vi "Timer Process.vi"(8 "error in (no error)":errorcluster, 10 "Timer Display Refnum":refnum<vi>, 11 "Background Control Queue":refnum<queue>) -> (0 "error out":errorcluster)   [LabVIEW 2015, in "Execution.lvclass"]
uses:
  Execution.lvclass
  BACKGROUND_CONTROL_MSG_TYPEDEF.ctl
panel:
  out "STOP_FLAG":bool
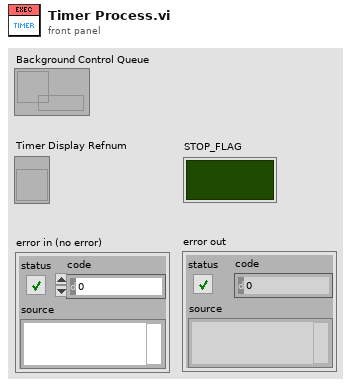
[diagram p1: front panel]
types:
  T1 = typedef "Execution.lvclass/BACKGROUND_CONTROL_MSG_TYPEDEF.ctl" = cluster{"Target":string, "Msg":string, "Data":variant}
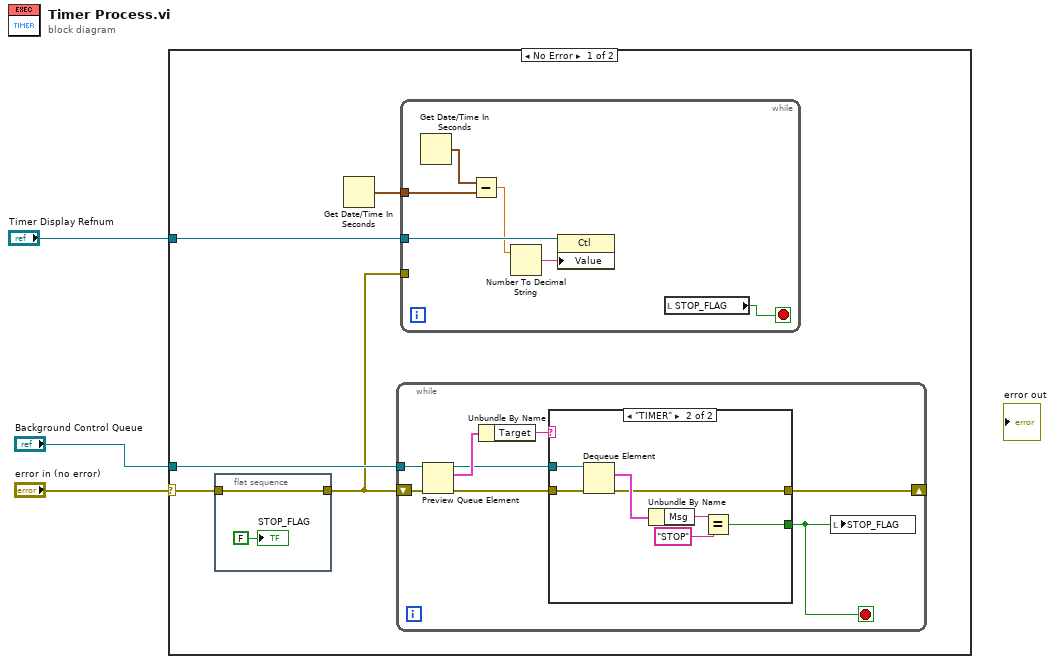
[diagram p0: block diagram]
diagram:
  n1 = case shown="No Error" "error in (no error)" {
    selector: "error in (no error)" -> [w6 _]
    tunnel: "Background Control Queue" -> [w7 _]
    tunnel: "Timer Display Refnum" -> [w4 _]
    frame No Error {
      n2 = flat-sequence {
        tunnel: w6 -> [w10]
        tunnel: [w10] -> w5
        frame #0 {
          "STOP_FLAG" <- FALSE ("STOP_FLAG")
        }
      }
      n3 = Get Date/Time In Seconds() -> (seconds since 1Jan1904=w8:timestamp)
      n4 = while {
        shift-right: [w12] -> _
        shift-left: w5 -> [w18]
        tunnel: w7 -> [w17]
        stop <- w11 stop-if-true
        n5 = Preview Queue Element(queue=w17, error in (no error)=w18) -> (queue out=w13:refnum<queue>, element=w16:T1, error out=w14:errorcluster)  [unwired: 1 in, 1 out]
        n6 = Unbundle By Name(w16) -> ("Target"=w15:string)
        n7 = case shown="\"TIMER\"" w15 {
          tunnel: w14 -> [w19 w26]
          tunnel: w13 -> [_ w25]
          tunnel: [w19 w23] -> w12
          tunnel: [_ w20] -> w11
          frame "False", Default {
          }
          frame "TIMER" {
            n8 = Dequeue Element(queue=w25, error in (no error)=w26) -> (element=w24:T1, error out=w23:errorcluster)  [unwired: 1 in, 2 out]
            n9 = Unbundle By Name(w24) -> ("Msg"=w22:string)
            n10 = Equal?(x=w22, y="STOP") -> (x = y?=w20:bool)
          }
        }
        n11 = local write "STOP_FLAG"(w11) -> ()
      }
      n12 = while {
        tunnel: w8 -> [w30]
        tunnel: w5 -> [_]
        tunnel: w4 -> [w29]
        stop <- w32 stop-if-true
        n13 = Get Date/Time In Seconds() -> (seconds since 1Jan1904=w31:timestamp)
        n14 = Subtract(x=w31, y=w30) -> (x-y=w28:dbl)
        n15 = Number To Decimal String(number=w28) -> (decimal integer string=w27:string)  [unwired: 1 in]
        n16 = property class="Ctl"(reference=w29, "Value"=w27) -> ()  [unwired: 1 in, 2 out]
        n17 = local read "STOP_FLAG"() -> (w32:bool)
      }
    }
    frame Error {
    }
  }
